vi "SwitchBoard_query.vi"(8 "error in":errorcluster, 10 "Buffer":string="MATRIX.TEMPERATURE", 11 "Handle":u32) -> (0 "error out":errorcluster, 2 "Read Buffer Out":string, 3 "Handle":u32)   [LabVIEW 2016]
panel:
  out "Bytes Read":u32
  out "Bytes Waiting":u32
  out "Bytes Written":u32
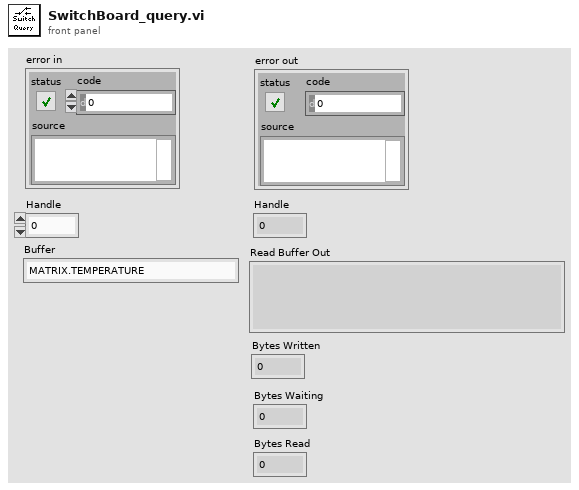
[diagram p1: front panel]
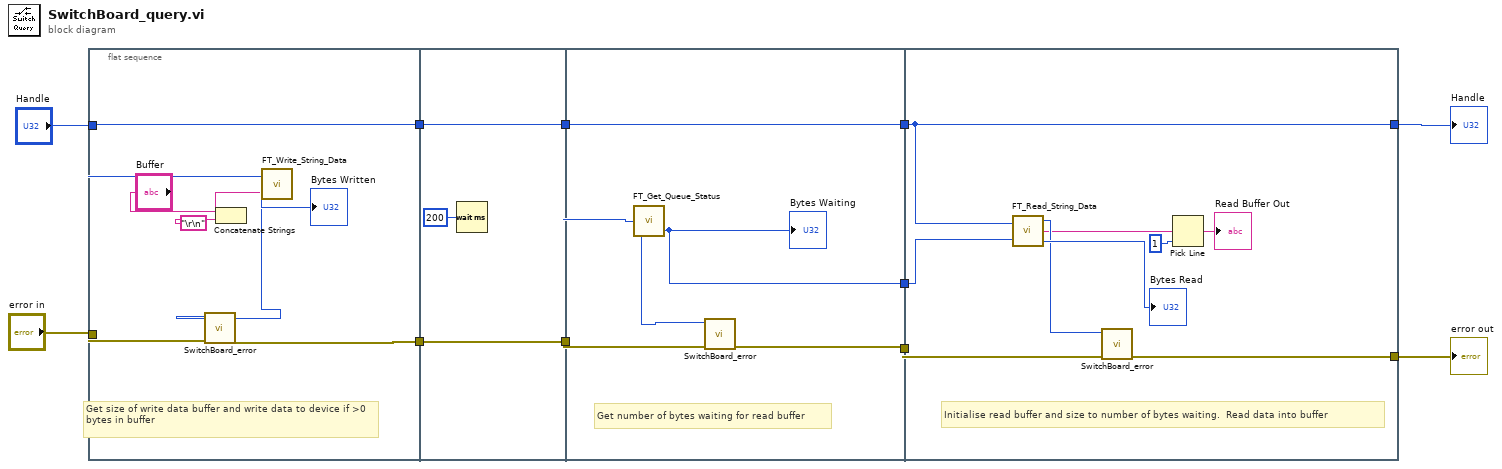
[diagram p0: block diagram]
diagram:
  n1 = flat-sequence {
    tunnel: [w15] -> w11
    tunnel: "Handle" -> [w15]
    tunnel: "error in" -> [w14]
    tunnel: [w12] -> w4
    tunnel: w11 -> [w22]
    tunnel: [w22] -> w10
    tunnel: w4 -> [w20]
    tunnel: [w20] -> w3
    tunnel: w10 -> [w27]
    tunnel: [w27] -> w9
    tunnel: [w26] -> w8
    tunnel: w3 -> [w25]
    tunnel: [w24] -> w2
    tunnel: w9 -> [w34]
    tunnel: w8 -> [w35]
    tunnel: [w34] -> w6
    tunnel: w2 -> [w33]
    tunnel: [w31] -> w1
    frame #0 {
      # "Get size of write data buffer and write data to device if >0 bytes in buffer"
      n2 = Concatenate Strings("Buffer", "\r\n") -> (w16:string)
      n3 = call "FT_Write_String_Data.vi"("Buffer"=w16, "Handle"=w15) -> ("Bytes Written"=→"Bytes Written":u32, "FT_Status"=w13:u32)
      n4 = call "SwitchBoard_error.vi"("error constant"=w14, "Code"=w13) -> ("error IO"=w12:errorcluster)  [unwired: 9 in]
    }
    frame #1 {
      n5 = Wait (ms)(milliseconds to wait=u32 200) -> ()  [unwired: 1 out]
    }
    frame #2 {
      # "Get number of bytes waiting for read buffer"
      n6 = call "FT_Get_Queue_Status.vi"("Handle"=w27) -> ("FT_Status"=w23:u32, "Bytes Waiting"=w26:u32)
      "Bytes Waiting" <- w26
      n7 = call "SwitchBoard_error.vi"("error constant"=w25, "Code"=w23) -> ("error IO"=w24:errorcluster)  [unwired: 9 in]
    }
    frame #3 {
      # "Initialise read buffer and size to number of bytes waiting.  Read data into buffer"
      n8 = call "FT_Read_String_Data.vi"("Handle"=w34, "Bytes To Read"=w35) -> ("FT_Status"=w32:u32, "Read Data"=w30:string, "Bytes Read"=→"Bytes Read":u32)
      n9 = call "SwitchBoard_error.vi"("error constant"=w33, "Code"=w32) -> ("error IO"=w31:errorcluster)  [unwired: 9 in]
      n10 = Pick Line(multi-line string=w30, line index=1) -> (output string=→"Read Buffer Out":string)  [unwired: 1 in]
    }
  }
  "Handle" <- w6
  "error out" <- w1
